vi "Configure SPI Clock.vi"(7 "Timeout (5e-7 s)":dbl=5e-07, 8 "error in (no error)":errorcluster, 9 "Clock Slope (0: Positive)":i32(ring) items=["Positive", "Rising", "Negative", "Falling"], 10 "Channel (1: Serial Bus 1)":i32(ring)=1 items=["Serial Bus 1"=1, "Serial Bus 2"=2, "Serial Bus 3"=3, "Serial Bus 4"=4], 11 "VISA resource name":refnum<visa-resource-name>) -> (0 "error out":errorcluster, 3 "VISA resource name out":refnum<visa-resource-name>)   [LabVIEW 2020, in "Agilent 90000 Series.lvlib"]
doc: "Configures the SPI serial clock."
uses:
  Agilent 90000 Series.lvlib
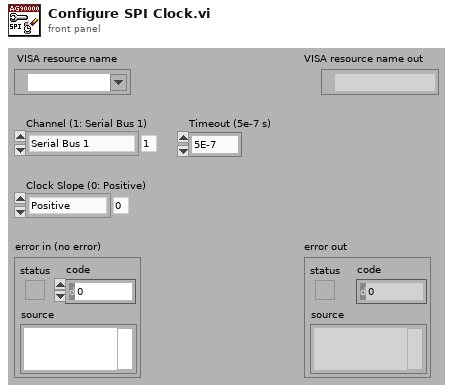
[diagram p1: front panel]
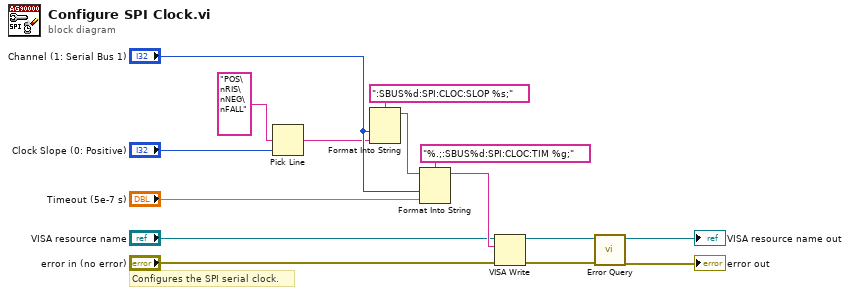
[diagram p0: block diagram]
diagram:
  # "Configures the SPI serial clock."
  n1 = Pick Line(multi-line string="POS\nRIS\nNEG\nFALL", line index="Clock Slope (0: Positive)") -> (output string=w11:string)  [unwired: 1 out]
  n2 = Format Into String(format string=":SBUS%d:SPI:CLOC:SLOP %s;", "Channel (1: Serial Bus 1)", w11) -> (resulting string=w10:string)  [unwired: 2 in, 1 out]
  n3 = Format Into String(format string="%.;:SBUS%d:SPI:CLOC:TIM %g;", initial string=w10, "Channel (1: Serial Bus 1)", "Timeout (5e-7 s)") -> (resulting string=w7:string)  [unwired: 1 in, 1 out]
  n4 = VISA Write(VISA resource name="VISA resource name", write buffer=w7, error in (no error)="error in (no error)") -> (VISA resource name out=w4:refnum<visa-resource-name>, error out=w3:errorcluster)  [unwired: 1 out]
  n5 = call "Error Query.vi"("error in (no error)"=w3, "VISA resource name"=w4) -> ("error out"=→"error out":errorcluster, "VISA resource name out"=→"VISA resource name out":refnum<visa-resource-name>)  [unwired: 8 out]
